vi "Face Recognizer.vi"() -> ()   [LabVIEW 2018]
uses:
  <vilib>/httpClient/LabVIEWHTTPClient.lvlib
panel:
  in  "Working directory":path=path "C:/Users/Mukund.S.SOLITONTECH/Desktop/SFR win"
  in  "stop":bool
  out "Json_data":string
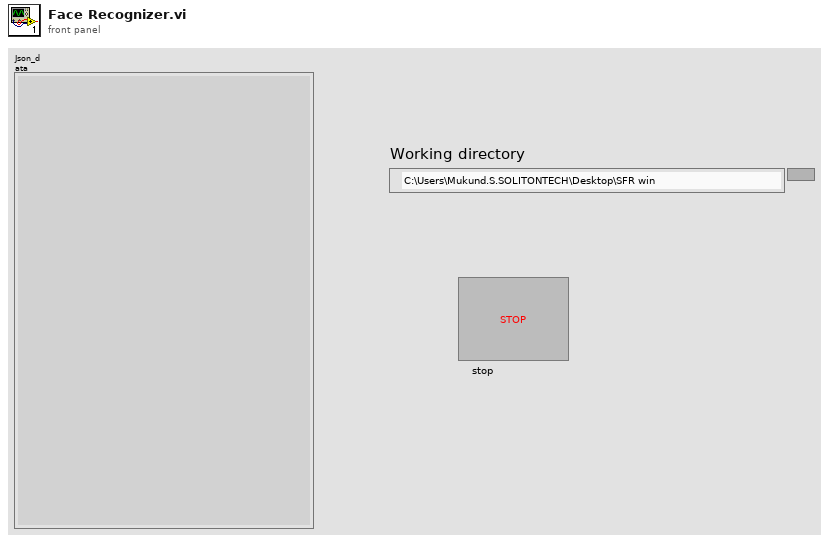
[diagram p1: front panel]
types:
  T1 = typedef "LabVIEWHTTPClient.lvlib/ClientHandle.ctl" = refnum<k1>
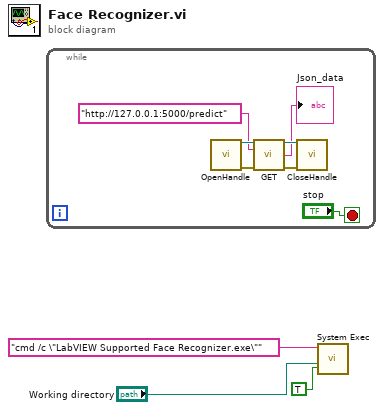
[diagram p0: block diagram]
diagram:
  n1 = while {
    stop <- "stop" stop-if-true
    n2 = call <vilib>:"OpenHandle.vi"() -> ("client handle out"=w10:T1, "error out"=w9:errorcluster)  [unwired: 14 in]
    n3 = call <vilib>:"GET.vi"("client handle"=w10, "url"="http://127.0.0.1:5000/predict", "error in (no error)"=w9) -> ("client handle out"=w8:T1, "body"=→"Json_data":string, "error out"=w7:errorcluster)  [unwired: 9 in, 1 out]
    n4 = call <vilib>:"CloseHandle.vi"("client handle"=w8, "error in (no error)"=w7) -> ()  [unwired: 13 in, 1 out]
  }
  n5 = call <vilib>:"System Exec.vi"("run minimized? (F)"=TRUE, "working directory"="Working directory", "command line"="cmd /c \"LabVIEW Supported Face Recognizer.exe\"") -> ()  [unwired: 5 in, 4 out]
